vi "logEventDetailedState.vi"(8 "error in (no error)":errorcluster, 10 "logevent_DetailedState_Ctl":T1, 11 "SALCommunicatorController in":refnum<class "SALCommunicatorController.lvclass">) -> (0 "error out":errorcluster, 3 "SALCommunicatorController out":refnum<class "SALCommunicatorController.lvclass">)   [LabVIEW 2016, in "SALCommunicatorController.lvclass"]
uses:
  SALCommunicatorController.lvclass
  ts_sallv_exa/DataTypes/logevent_DetailedState.ctl
  ts_sallv_exa/SALLV_EXA.lvlib
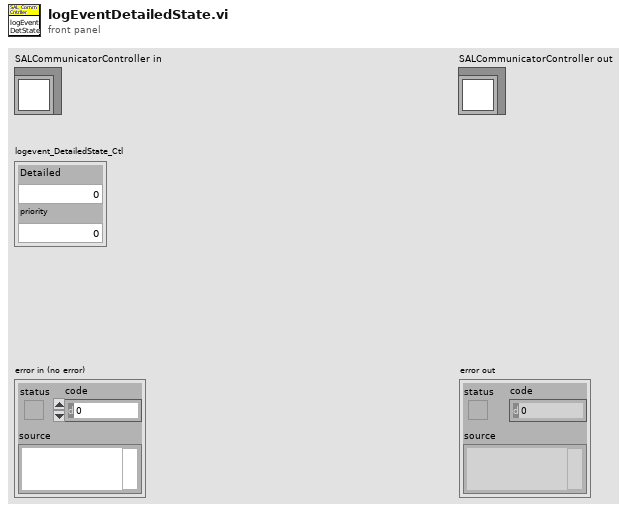
[diagram p1: front panel]
types:
  T1 = typedef "SALLV_EXA.lvlib/logevent_DetailedState.ctl" = cluster{"Detailed":u16, "priority":i32}
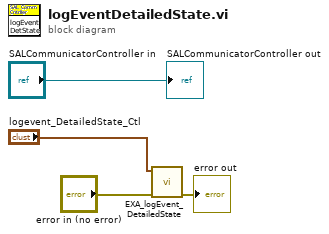
[diagram p0: block diagram]
diagram:
  n1 = call "EXA_logEvent_DetailedState.vi"("error in (no error)"="error in (no error)", "logevent_DetailedState_Ctl"="logevent_DetailedState_Ctl") -> ("error out"=→"error out":errorcluster)  [unwired: 7 in, 2 out]
  "SALCommunicatorController out" <- "SALCommunicatorController in"
